vi "GlobalLock.vi"(6 "GL Functions":T1, 8 "error in (no error)":errorcluster, 11 "CData In":refnum<class "CData.lvclass">) -> (0 "error out":errorcluster, 2 "Locked?":bool, 3 "CData Out":refnum<class "CData.lvclass">)   [LabVIEW 2014]
uses:
  Controls/GL Functions.ctl
  StateStore/Class/CData.lvclass
panel:
  # "Global Lock"
  # "INPUTS"
  # "OUTPUTS"
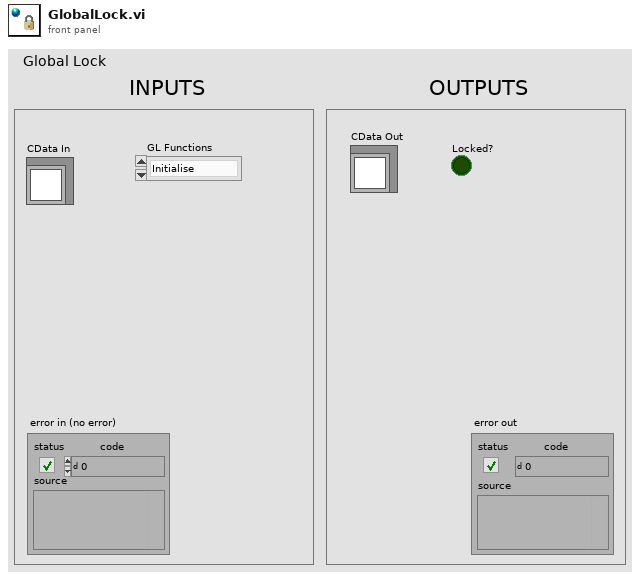
[diagram p1: front panel]
types:
  T1 = typedef "GL Functions.ctl" = enum16{"Initialise", "Get", "Set", "Dispose", "Query"}
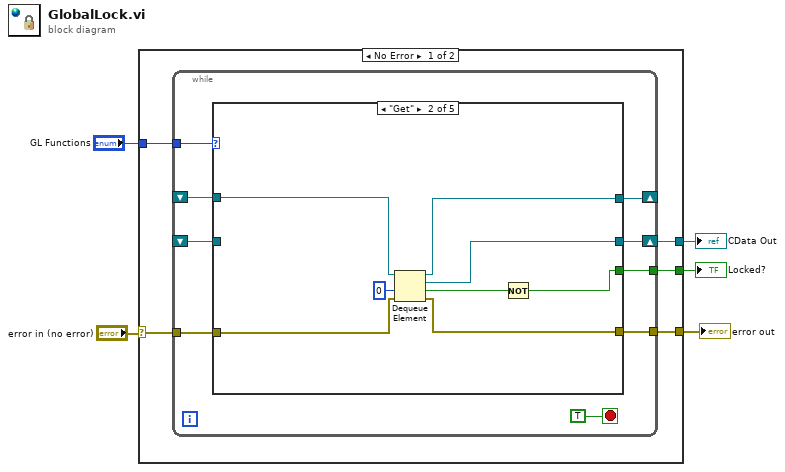
[diagram p0: block diagram]
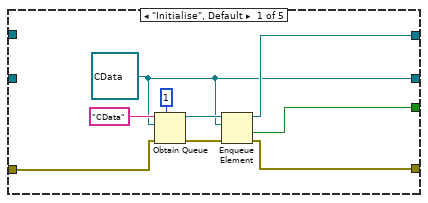
[diagram p2: hidden frame]
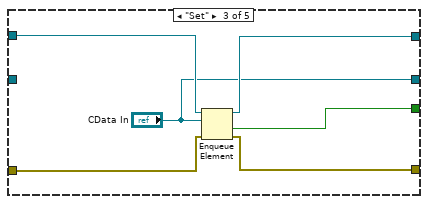
[diagram p3: hidden frame]
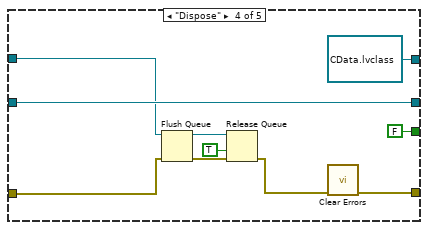
[diagram p4: hidden frame]
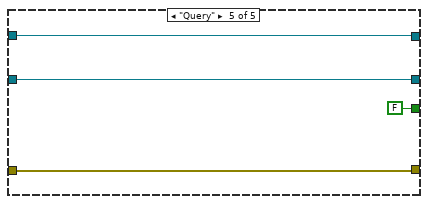
[diagram p5: hidden frame]
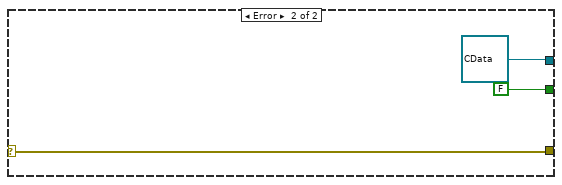
[diagram p6: hidden frame]
diagram:
  n1 = case shown="No Error" "error in (no error)" {
    selector: "error in (no error)" -> [w9 w59]
    tunnel: "GL Functions" -> [w10 _]
    tunnel: [w8 w59] -> w3
    tunnel: [w7 FALSE ("timed out?")] -> w2
    tunnel: [w6 refnum<class "CData.lvclass"> refnum ("CData In")] -> w1
    frame No Error {
      n2 = while {
        tunnel: w10 -> [w18]
        tunnel: w9 -> [w17]
        shift-right: [w16] -> w6
        shift-left: _ -> [w12]
        tunnel: [w15] -> w8
        shift-right: [w14] -> _
        shift-left: _ -> [w13]
        tunnel: [w11] -> w7
        stop <- TRUE stop-if-true
        n3 = case shown="\"Get\"" w18 {
          tunnel: w17 -> [w25 w36 w42 w46 w54]
          tunnel: [w21 w32 "CData In" w51 w56] -> w16
          tunnel: [w26 w35 w41 w44 w54] -> w15
          tunnel: [w24 w33 w39 refnum<queue> refnum ("queue out") w55] -> w14
          tunnel: w13 -> [_ w34 w40 w47 w55]
          tunnel: w12 -> [_ _ _ w51 w56]
          tunnel: [w20 w30 w37 FALSE ("timed out?") FALSE ("timed out?")] -> w11
          frame "Initialise", Default {
            w21 = refnum<class "CData.lvclass"> refnum ("CData.lvclass")
            n4 = Obtain Queue(max queue size (-1, unlimited)=1, name (unnamed)="CData", element data type=w21, error in (no error)=w25) -> (queue out=w23:refnum<queue>, error out=w27:errorcluster)  [unwired: 1 in, 1 out]
            n5 = Enqueue Element(queue=w23, element=w21, error in (no error)=w27) -> (queue out=w24:refnum<queue>, timed out?=w20:bool, error out=w26:errorcluster)  [unwired: 1 in]
          }
          frame "Get" {
            n6 = Dequeue Element(queue=w34, timeout in ms (-1)=0, error in (no error)=w36) -> (queue out=w33:refnum<queue>, element=w32:refnum<class "CData.lvclass">, timed out?=w31:bool, error out=w35:errorcluster)
            n7 = Not(x=w31) -> (.not. x?=w30:bool)
          }
          frame "Set" {
            n8 = Enqueue Element(queue=w40, element="CData In", error in (no error)=w42) -> (queue out=w39:refnum<queue>, timed out?=w37:bool, error out=w41:errorcluster)  [unwired: 1 in]
          }
          frame "Dispose" {
            n9 = Flush Queue(queue=w47, error in (no error)=w46) -> (queue out=w48:refnum<queue>, error out=w50:errorcluster)  [unwired: 1 out]
            n10 = Release Queue(queue=w48, force destroy? (F)=TRUE, error in (no error)=w50) -> (error out=w45:errorcluster)  [unwired: 2 out]
            n11 = call <vilib>:"Clear Errors.vi"("error in (no error)"=w45) -> ("error out"=w44:errorcluster)  [unwired: 5 in, 1 out]
          }
          frame "Query" {
          }
        }
      }
    }
    frame Error {
    }
  }
  "error out" <- w3
  "Locked?" <- w2
  "CData Out" <- w1
